vi "PH_Cont-601k_PSU.evt Call Charge.vi"(0 "i ref in":refnum<vi>, 1 "Instance name":string="N/A", 5 "error in":errorcluster) -> (14 "i ref out":refnum<vi>, 19 "error out":errorcluster)   [LabVIEW 2014, in "PH_Cont-601k_PSU.lvlib"]
doc: "This VI calls an event by a simple call."
uses:
  PH_Cont-601k_PSU.lvlib
  CSCore/BaseProcess/BaseProcess.lvlib
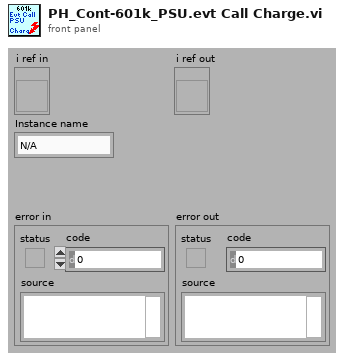
[diagram p1: front panel]
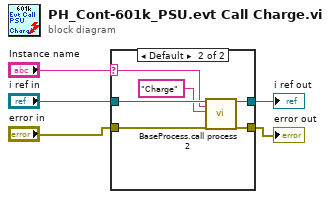
[diagram p0: block diagram]
diagram:
  n1 = case shown="Default" "Instance name" {
    selector: "Instance name" -> [_ w9]
    tunnel: [w6 w13] -> w5
    tunnel: "error in" -> [w6 w12]
    tunnel: [w7 w11] -> w2
    tunnel: "i ref in" -> [w7 w10]
    frame "", "N/A" {
    }
    frame Default {
      n2 = call "BaseProcess.call process 2.vi"("i ref in"=w10, "Object"=w9, "Selector"="Charge", "error in (no error)"=w12) -> ("i ref out"=w11:refnum<vi>, "error out"=w13:errorcluster)  [unwired: 14 in]
    }
  }
  "error out" <- w5
  "i ref out" <- w2
